vi "Relay switch.vi"() -> ()   [LabVIEW 2009]
panel:
  in  "stop":bool
  in  "Switch Time":dbl[unit]
  in  "Pulse Length":dbl[unit]
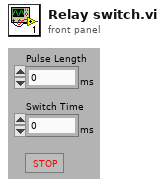
[diagram p1: front panel]
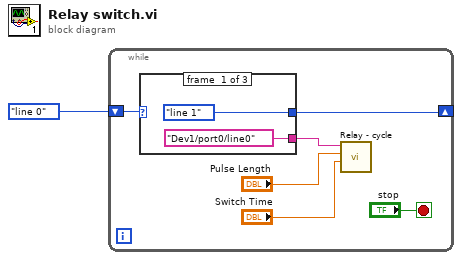
[diagram p0: block diagram]
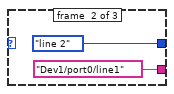
[diagram p2: hidden frame]
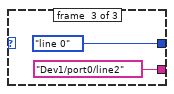
[diagram p3: hidden frame]
diagram:
  n1 = while {
    shift-right: [w2] -> _
    shift-left: enum16{"line 0", "line 1", "line 2"}."line 0" ("line") -> [w4]
    stop <- "stop" stop-if-true
    n2 = case shown="\"line 2\"" w4 {
      tunnel: [enum16{"line 0", "line 1", "line 2"}."line 1" ("line") enum16{"line 0", "line 1", "line 2"}."line 2" ("line") enum16{"line 0", "line 1", "line 2"}."line 0" ("line")] -> w2
      tunnel: [tag "Dev1/port0/line0" ("lines") tag "Dev1/port0/line1" ("lines") tag "Dev1/port0/line2" ("lines")] -> w3
      frame #0 {
      }
      frame #1 {
      }
      frame #2 {
      }
    }
    n3 = call "Relay - cycle.vi"("switch time"="Switch Time", "pulse length"="Pulse Length", "task in"=w3) -> ()  [unwired: 1 in, 8 out]
  }
